vi "StepWait.vi"(7 "Time to wait":string, 11 "error in":errorcluster) -> (8 "Results":T1, 15 "error out":errorcluster)   [LabVIEW 2021]
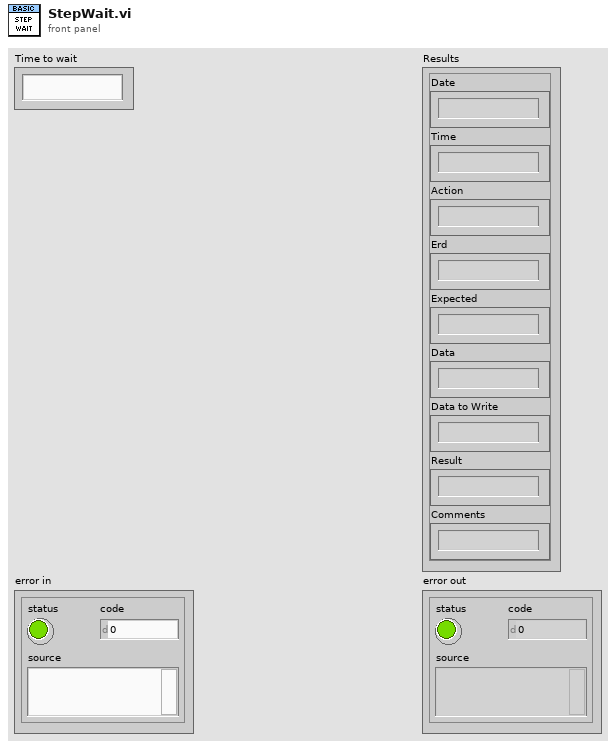
[diagram p1: front panel]
types:
  T1 = cluster{"Date":string, "Time":string, "Action":string, "Erd":string, "Expected":string, "Data":string, "Data to Write":string, "Result":string, "Comments":string}
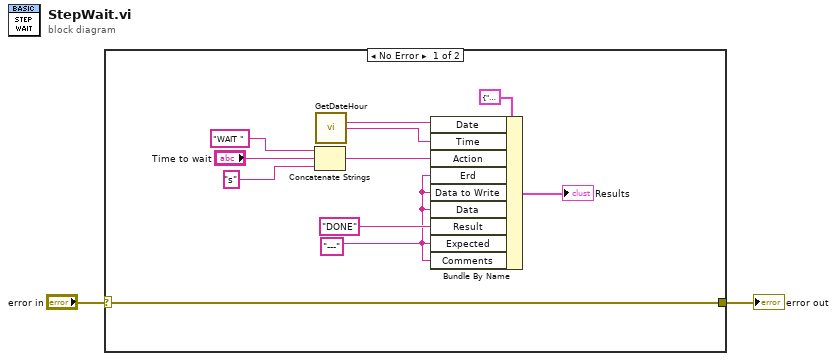
[diagram p0: block diagram]
diagram:
  n1 = case shown="No Error" "error in" {
    selector: "error in" -> [w3 w14]
    tunnel: [w3 w14] -> w1
    frame No Error {
      w4 = "---"
      n2 = Concatenate Strings("WAIT " ("string"), "Time to wait", "s" ("string")) -> (w5:string)
      n3 = call "GetDateHour.vi"() -> ("Date"=w12:string, "Hour"=w11:string)  [unwired: 14 in]
      n4 = Bundle By Name(cluster=T1 {"Date"="", "Time"="", "Action"="", "Erd"="", "Expected"="", "Data"="", "Data to Write"="", "Result"="", "Comments"=""}, "Date"=w12, "Time"=w11, "Action"=w5, "Erd"=w4, "Data to Write"=w4, "Data"=w4, "Result"="DONE", "Expected"=w4, "Comments"=w4) -> (→"Results":T1)
    }
    frame Error {
    }
  }
  "error out" <- w1
